vi "DAQmx Write (Digital Wfm 1Chan 1Samp).vi"(0 "task/channels in":refnum<k21>, 1 "auto start":bool=TRUE, 7 "data":digitalwaveform(waveform)={"t0"=timestamp(0 s since 1904-01-01), "dt"=0.0, "Y"={"transitions"=[], "data"=[]}, "error"={"status"=FALSE, "code"=37421928, "source"=""}}, 9 "timeout":dbl=10.0 format="%0.2f", 11 "error in":errorcluster) -> (4 "task out":refnum<k21>, 10 "number of samples written per channel":u32, 15 "error out":errorcluster)   [LabVIEW 2024]
doc: "Writes a digital waveform that contains a single sample to a task that contains a single digital output channel."
uses:
  nilvaiu.dll
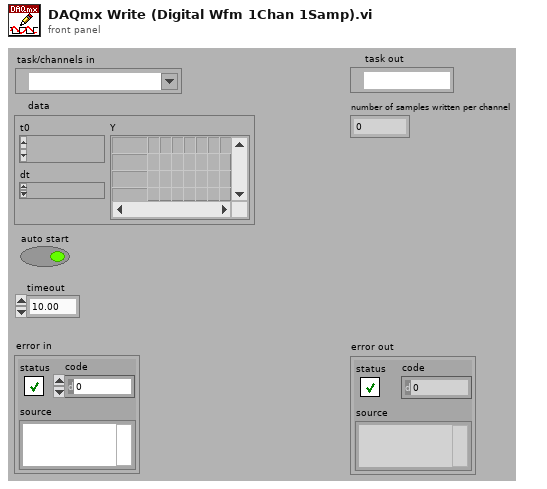
[diagram p1: front panel]
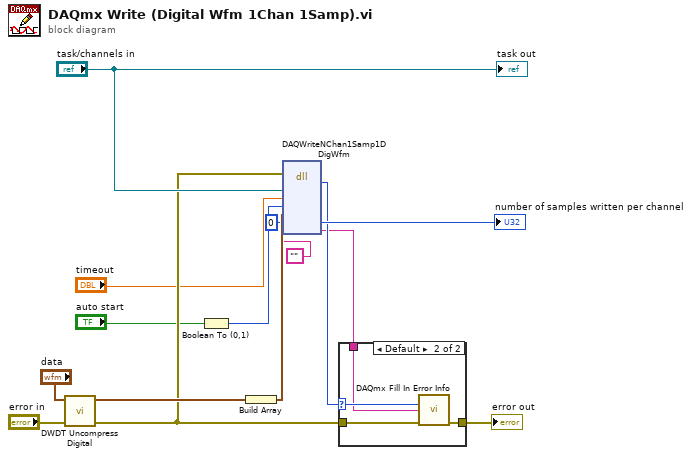
[diagram p0: block diagram]
diagram:
  n1 = call "DWDT Uncompress Digital.vi"("error in (no error)"="error in", "compressed digital waveform"="data") -> ("error out"=w10:errorcluster, "uncompressed digital waveform"=w11:digitalwaveform)  [unwired: 8 out]
  n2 = Boolean To (0,1)(Boolean="auto start") -> (0, 1=w5:i16)
  n3 = Build Array(w11) -> (w4:digitalwaveform[])
  n4 = dll-call lib="nilvaiu.*" fn="DAQWriteNChan1Samp1DDigWfm"(error in=w10, "taskID"="task/channels in", "timeout"="timeout", "autoStart"=w5, "data"=w4, "nunmSamplesWriten"=u32 0, "extendedErrorInfo"="") -> (w6:i32, "nunmSamplesWriten"=→"number of samples written per channel":u32, "extendedErrorInfo"=w2:string)  [unwired: 4 in, 4 out]
  n5 = case shown="Default" w6 {
    selector: w6 -> [_ w18]
    tunnel: w10 -> [w16 w20]
    tunnel: [w16 w19] -> w14
    tunnel: w2 -> [_ w17]
    frame 0 {
    }
    frame Default {
      n6 = call "DAQmx Fill In Error Info.vi"("status code"=w18, "extended error info"=w17, "error in"=w20) -> ("error out"=w19:errorcluster)  [unwired: 1 in, 11 out]
    }
  }
  "error out" <- w14
  "task out" <- "task/channels in"
